vi "Global Variables.vi"() -> ()   [LabVIEW 2016]
panel:
  out "z+y- last state":bool
  out "z-y+ last state":bool
  out "z-y- last state":bool
  out "z+y+ last state":bool
  out "y- last state":bool
  out "y+ last state":bool
  out "z- last state":bool
  out "z+ last state":bool
  out "- last state":bool
  out "+ last state":bool
  in  "Ressolution Codeur":dbl
  in  "Pulse/Degre":dbl
  in  "Diametre Galet Codeur":dbl
  in  "Diametre Plateau":dbl
  in  "Decel Max":dbl
  in  "Accel Max":dbl
  in  "MaxSpeed":dbl
  in  "Decel":dbl
  in  "Accel":dbl
  # "User Settings"
  # "System settings"
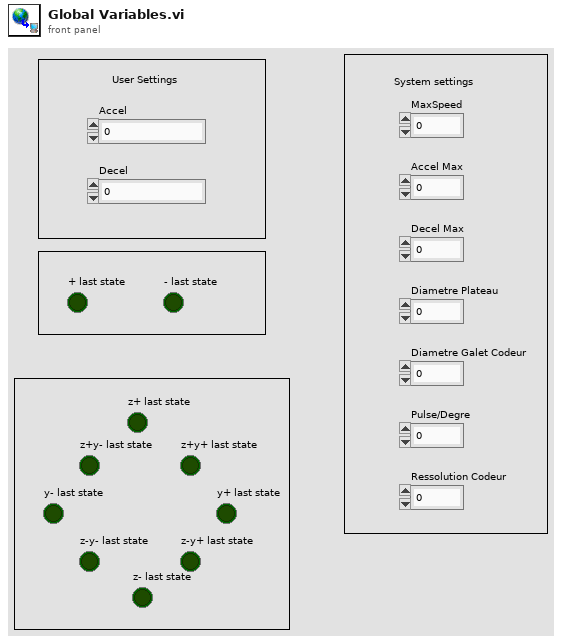
[diagram p1: front panel]
diagram:
